vi "Icon.vi"(11 "Caraya Item in":refnum<class "Caraya Item.lvclass">) -> (2 "Icon":T1 caption="Icon (16x16 px)")   [LabVIEW 2019, in "Caraya Library.lvlib" / "Caraya Item.lvclass"]
uses:
  Caraya Item.lvclass
  libs/Solution.lvlibp/1abvi3w/vi.lib/picture/picture.llb/imagedata.ctl
  libs/Solution.lvlibp
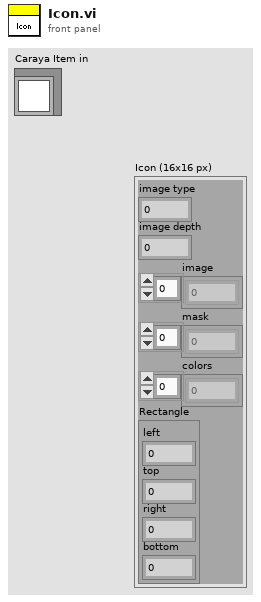
[diagram p1: front panel]
types:
  T1 = typedef "Solution.lvlibp/imagedata.ctl" = cluster{"image type":i32, "image depth":i32, "image":u8[], "mask":u8[], "colors":u32[], "Rectangle":cluster{"left":i16, "top":i16, "right":i16, "bottom":i16}}
  T2 = typedef "imagedata.ctl" = cluster{"image type":i32, "image depth":i32, "image":u8[], "mask":u8[], "colors":u32[], "Rectangle":cluster{"left":i16, "top":i16, "right":i16, "bottom":i16}}
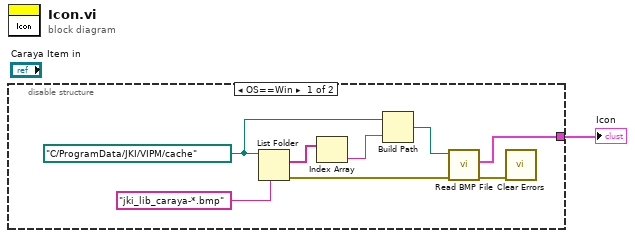
[diagram p0: block diagram]
diagram:
  n1 = disable-structure shown="OS==Win" {
    disable-tunnel: [w2 _] -> w1
    frame condition #0 (active) {
      w6 = path "C:/ProgramData/JKI/VIPM/cache"
      n2 = List Folder(path=w6, pattern="jki_lib_caraya-*.bmp") -> (filenames=w8:string[], error out=w5:errorcluster)  [unwired: 2 in, 2 out]
      n3 = Index Array(array=w8) -> (element=w7:string)  [unwired: 1 in]
      n4 = Build Path(base path=w6, name or relative path=w7) -> (appended path=w3:path)
      n5 = call <vilib>:"Read BMP File.vi"("error in (no error)"=w5, "path to BMP file"=w3) -> ("error out"=w4:errorcluster, "image data"=w2:T2)  [unwired: 7 in, 1 out]
      n6 = call <vilib>:"Clear Errors.vi"("error in (no error)"=w4) -> ()  [unwired: 5 in, 2 out]
    }
    frame condition #1 {
    }
  }
  "Icon" <- w1
